vi "Get Last Run Scan XML Settings Path.vi"(8 "error in (no error)":errorcluster) -> (0 "error out":errorcluster, 2 "scanreader path out":path, 3 "XML path out":path)   [LabVIEW 2017]
uses:
  Global/File Locations.vi
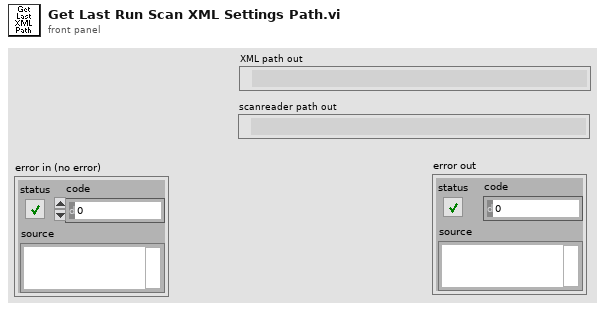
[diagram p1: front panel]
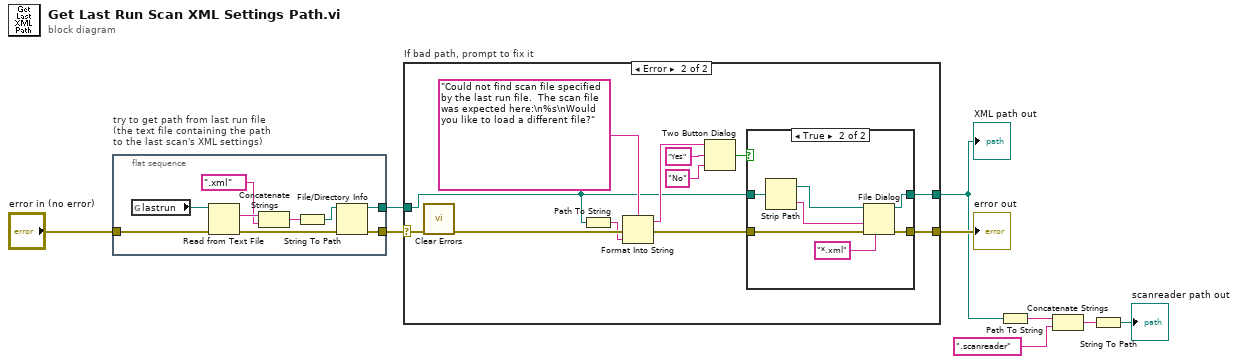
[diagram p0: block diagram]
diagram:
  n1 = flat-sequence "try to get path from last run file\n(the text file containing the path\nto the last scan's XML settings)" {
    tunnel: "error in (no error)" -> [w17]
    tunnel: [w15] -> w7
    tunnel: [w10] -> w9
    frame #0 {
      n2 = global read "File Locations.vi" "lastrun"() -> (w18:path)
      n3 = Read from Text File(file (use dialog)=w18, error in=w17) -> (text=w14:string, error out=w16:errorcluster)  [unwired: 4 out]
      n4 = Concatenate Strings(w14, ".xml") -> (w13:string)
      n5 = String To Path(string=w13) -> (path=w11:path)
      n6 = File/Directory Info(path=w11, error in=w16) -> (path out=w10:path, error out=w15:errorcluster)  [unwired: 5 out]
    }
  }
  n7 = case "If bad path, prompt to fix it" shown="Error" w7 {
    selector: w7 -> [w20 w27]
    tunnel: [w19 w29] -> w5
    tunnel: [w20 w28] -> w8
    tunnel: w9 -> [w19 w21]
    frame No Error {
    }
    frame Error {
      n8 = call <vilib>:"Clear Errors.vi"("error in (no error)"=w27) -> ("error out"=w25:errorcluster)  [unwired: 1 in, 5 out]
      n9 = Path To String(path=w21) -> (string=w23:string)
      n10 = Format Into String(format string="Could not find scan file specified by the last run file.  The scan file was expected here:\n%s\nWould you like to load a different file?", error in=w25, w23) -> (resulting string=w22:string, error out=w24:errorcluster)  [unwired: 1 in]
      n11 = Two Button Dialog(message=w22, 1:"No", 2:"Yes") -> (T button?=w30:bool)
      n12 = case shown="True" w30 {
        tunnel: [w33 w41] -> w29
        tunnel: w24 -> [w34 w38]
        tunnel: [w34 w37] -> w28
        tunnel: w21 -> [w33 w35]
        frame False {
        }
        frame True {
          n13 = Strip Path(path=w35) -> (stripped path=w40:path, name=w39:string)
          n14 = File Dialog(6:"*.xml" ("pattern (all files)"), 8:w38, 9:w39, 11:w40) -> (0:w37:errorcluster, 3:w41:path)  [unwired: 5 out]
        }
      }
    }
  }
  "XML path out" <- w5
  "error out" <- w8
  n15 = Path To String(path=w5) -> (string=w4:string)
  n16 = Concatenate Strings(w4, ".scanreader" ("string")) -> (w2:string)
  n17 = String To Path(string=w2) -> (path=→"scanreader path out":path)
